vi "PH_ImageOperator.write PSDB Trace data.vi"(0 "i ref in":refnum<vi>, 5 "error in":errorcluster) -> (14 "i ref out":refnum<vi>, 15 "Trace Boolean data":T5[](array[typedef]), 16 "Trace Numeric data":T4[](array[typedef]), 17 "Trace 2D data":T3[](array[typedef]), 18 "Trace String data":T1[](array[typedef]), 19 "error out":errorcluster)   [LabVIEW 2014, in "PH_ImageOperator.lvlib"]
uses:
  PH_ImageOperator.lvlib
  PH_Basics/PH_PSDBWriter/PH_PSDBWriter.Boolean dataset.ctl
  PH_Basics/PH_PSDBWriter/PH_PSDBWriter.Numeric dataset.ctl
  PH_Basics/PH_PSDBWriter/PH_PSDBWriter.2D dataset.ctl
  CSlibraries-extern/psdb_lv/PSDB_AxisDescription.ctl
  PH_Basics/PH_PSDBWriter/PH_PSDBWriter.String dataset.ctl
  PH_Basics/PH_StatusHandler/PH_StatusHandler.Status.ctl
  CSlibraries-extern/psdb_lv/PSDB.lvlib
  PH_Basics/PH_PSDBWriter/PH_PSDBWriter.lvlib
  PH_Basics/PH_StatusHandler/PH_StatusHandler.lvlib
panel:
  in  "axis description":T2
  in  "2D data":T3
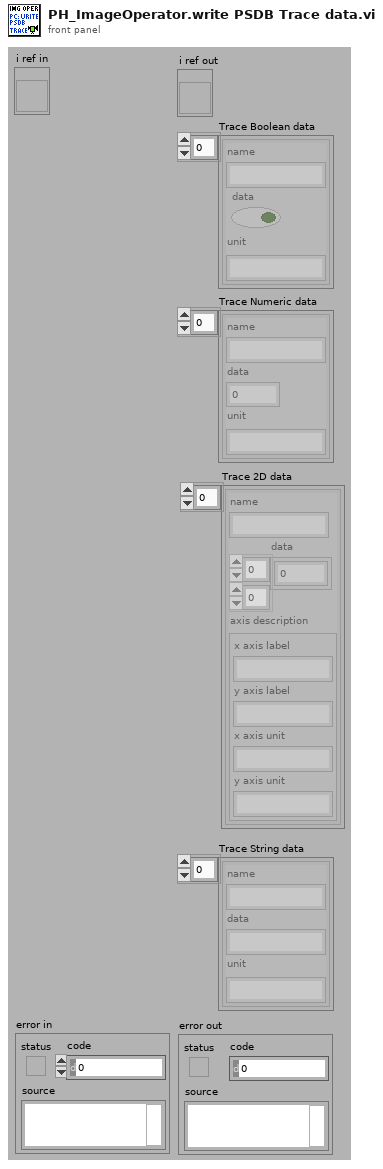
[diagram p1: front panel]
types:
  T1 = typedef "PH_PSDBWriter.lvlib/PH_PSDBWriter.String dataset.ctl" = cluster{"name":string, "data":string, "unit":string}
  T2 = typedef "PSDB.lvlib/PSDB_AxisDescription.ctl" = cluster{"x axis label":string, "y axis label":string, "x axis unit":string, "y axis unit":string}
  T3 = typedef "PH_PSDBWriter.lvlib/PH_PSDBWriter.2D dataset.ctl" = cluster{"name":string, "data":dbl[][], "axis description":T2}
  T4 = typedef "PH_PSDBWriter.lvlib/PH_PSDBWriter.Numeric dataset.ctl" = cluster{"name":string, "data":dbl, "unit":string}
  T5 = typedef "PH_PSDBWriter.lvlib/PH_PSDBWriter.Boolean dataset.ctl" = cluster{"name":string, "data":bool, "unit":string}
  T6 = typedef "PH_ImageOperator.lvlib/PH_ImageOperator.i attribute.ctl" = cluster{"GUI Refs":cluster{"Delete":refnum<vi>, "Calibration status":refnum<vi>, "BI subtracted":refnum<vi>, "calc Energy":refnum<vi>, "Energy: expected value":refnum<vi>, "Energy: Tolerance":refnum<vi>, "Energy calculated":refnum<vi>, "Energy":refnum<vi>, "calc Beam Anal":refnum<vi>, "Maj Diam 1/esquare":refnum<vi>, "Min Diam 1/esquare":refnum<vi>, "Azi Angle":refnum<vi>, "Min/Maj Diam esquare":refnum<vi>, "Beam analysed":refnum<vi>, "CoG - x":refnum<vi>, "CoG - y":refnum<vi>, "BA: Method":refnum<vi>, "BA: Steps":refnum<vi>, "BA: Factor":refnum<vi>, "calc Traces":refnum<vi>, "Traces: Fit Gauss":refnum<vi>, "Traces calculated":refnum<vi>, "Maj FWHM":refnum<vi>, "Min FWHM":refnum<vi>, "Major Trace":refnum<vi>, "Minor Trace":refnum<vi>, "Maj Fit Order":refnum<vi>, "Min Fit Order":refnum<vi>, "Position calculated":refnum<vi>, "Position":refnum<vi>, "Type":refnum<vi>, "Center":refnum<vi>, "exp - X":refnum<vi>, "exp - Y":refnum<vi>, "Tolerance":refnum<vi>, "f":refnum<vi>, "M":refnum<vi>, "D":refnum<vi>, "q":refnum<vi>, "Dummy Method":refnum<vi>, "Dummy Type":refnum<vi>, "Global On":refnum<vi>, "Traces: No offset":refnum<vi>, "Maj 99%":refnum<vi>, "Min 99%":refnum<vi>, "GUI FF Image":refnum<vi>, "calc Fill Factor":refnum<vi>, "FF calculated":refnum<vi>, "Fill Factor: Filter?":refnum<vi>, "FF: Damage Threshold":refnum<vi>, "FF: Threshold":refnum<vi>, "FF: max allow. Energy":refnum<vi>, "FF: Fillfactor":refnum<vi>, "Calibration data":refnum<vi>}, "List of GUIs":string[], "Calibration":cluster{"Status":T7, "Calibration data":T8, "Calibration Data File":path}, "Final Image":cluster{"BI Subtraction Failure":bool}, "Energy":cluster{"on":bool, "expected value [mJ]":dbl, "Tolerance [%]":dbl, "State":T7, "Energy [mJ]":dbl, "Unit":string, "calculated @":timestamp}, "Beam Analysis":cluster{"on":bool, "Data":T9, "Method":bool, "Steps":i32, "Factor":i32, "ROI":cluster{"Left":i32, "Top":i32, "Right":i32, "Bottom":i32}, "analysed @":timestamp}, "Trace Analysis":cluster{"on":bool, "Fit on":bool, "Maj FWHM":dbl, "Min FWHM":dbl, "Maj Fit Order":i32, "Min Fit Order":i32, "No Offset":bool, "Maj 99%":dbl, "Min 99%":dbl, "Traces":cluster{"XScaleName":string, "Y Scale Minimum":sgl, "Y Scale Maximum":sgl, "X Scale Minimum":sgl, "X Scale Maximum":sgl, "Traces":cluster{"Index":sgl[], "Trace":dbl[]}[]}[], "analysed @":timestamp}, "Position Analysis":cluster{"on":bool, "exp - X":i32, "exp - Y":i32, "focal length [mm]":dbl, "Magnification":dbl, "Delta":dbl, "Theta":dbl, "Tolerance":dbl, "Type":bool, "analysed @":timestamp}, "Fill Factor":cluster{"on":bool, "Filter on?":bool, "Threshold":dbl, "Damage Threshold [J/cm²]":dbl, "Fillfactor":dbl, "Max. allowed Energy [J]":dbl, "calculated @":timestamp}, "Statistician Service ID":i32, "Images":cluster{"Background":T10, "OP":T10, "GUI":T10, "BA: ROI":T10, "Trace: Turn":T10, "FF: Main":T10, "FF: Help":T10, "PSDB: BG":T10, "PSDB: OP":T10, "PSDB: FF":T10}}
  T7 = typedef "PH_StatusHandler.lvlib/PH_StatusHandler.Status.ctl" = i16
  T8 = typedef "PH_ImageCalibrator.lvlib/PH_ImageCalibrator.Calibration Data.ctl" = cluster{"Date":string, "Time":string, "Cam Settings":cluster{"Cam ID":string, "Gain":dbl, "Brightness":dbl, "Shutter":dbl, "Cam Error":bool, "Mode":i32}, "Background Image":cluster{"Image":dbl[][], "Image Error":bool}, "Linear Calibration":cluster{"Calibration Factor":dbl, "not mm or mrad":bool}, "Energy Calibration":cluster{"Calibration Factor":dbl, "no mJ":bool}}
  T9 = typedef "PH_ImageOperator.lvlib/PH_ImageOperator.Beam Analysis Data.ctl" = cluster{"CoG-x":sgl, "CoG-y":sgl, "Maj Dim":dbl, "Min Dim":dbl, "Ellipticity":dbl, "Azimuth Angle [rad]":dbl, "Azi Angle rel to Maj?":bool}
  T10 = typedef "IMAQ Image.ctl" = refnum<image>
  T11 = cluster{"XScaleName":string, "Y Scale Minimum":sgl, "Y Scale Maximum":sgl, "X Scale Minimum":sgl, "X Scale Maximum":sgl, "Traces":cluster{"Index":sgl[], "Trace":dbl[]}[]}[]
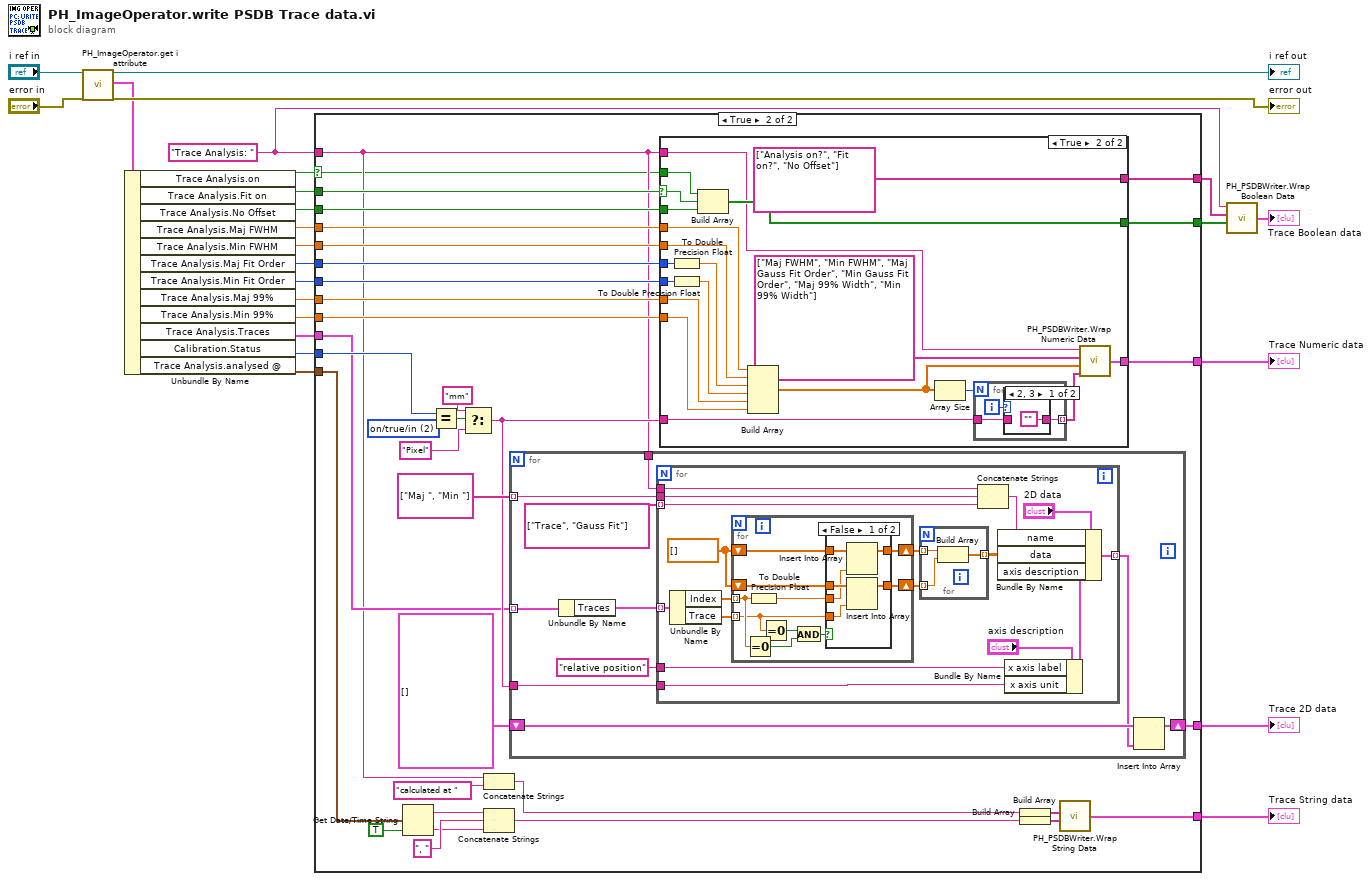
[diagram p0: block diagram]
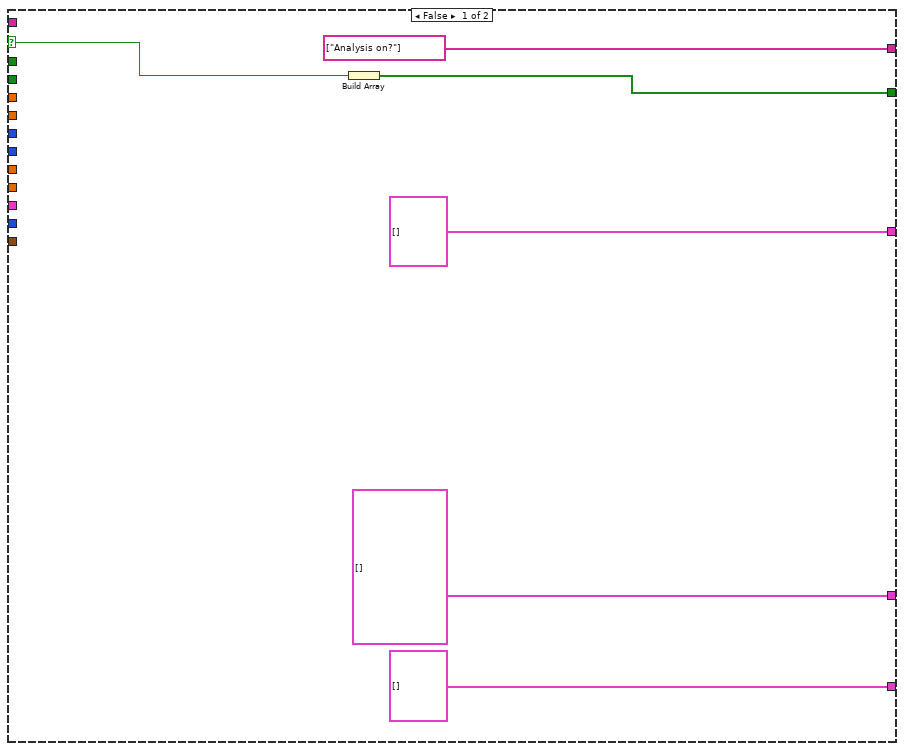
[diagram p2: hidden frame]
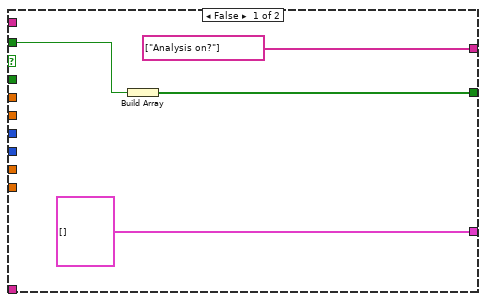
[diagram p3: hidden frame]
diagram:
  w2 = "Trace Analysis: " ("string")
  n1 = call "PH_ImageOperator.get i attribute.vi"("i ref in"="i ref in", "error in (no error)"="error in") -> ("i ref out"=→"i ref out":refnum<vi>, "i attribute"=w14:T6, "error out"=→"error out":errorcluster)  [unwired: 15 in]
  n2 = Unbundle By Name(w14) -> ("Trace Analysis.on"=w8:bool, "Trace Analysis.Fit on"=w7:bool, "Trace Analysis.No Offset"=w9:bool, "Trace Analysis.Maj FWHM"=w20:dbl, "Trace Analysis.Min FWHM"=w19:dbl, "Trace Analysis.Maj Fit Order"=w18:i32, "Trace Analysis.Min Fit Order"=w17:i32, "Trace Analysis.Maj 99%"=w16:dbl, "Trace Analysis.Min 99%"=w15:dbl, "Trace Analysis.Traces"=w12:T11, "Calibration.Status"=w13:T7, "Trace Analysis.analysed @"=w6:timestamp)
  n3 = case shown="True" w8 {
    selector: w8 -> [w26 w37]
    tunnel: w20 -> [_ w64]
    tunnel: w19 -> [_ w63]
    tunnel: w18 -> [_ w62]
    tunnel: w17 -> [_ w61]
    tunnel: w16 -> [_ w60]
    tunnel: w15 -> [_ w59]
    tunnel: w13 -> [_ w58]
    tunnel: w12 -> [_ w40]
    tunnel: [T3[] [] ("Trace 2D data") w52] -> w11
    tunnel: [T4[] [] w49] -> w10
    tunnel: w9 -> [_ w48]
    tunnel: w7 -> [_ w47]
    tunnel: w6 -> [_ w42]
    tunnel: [T1[] [] w33] -> w5
    tunnel: w2 -> [_ w39]
    tunnel: [w25 w38] -> w4
    tunnel: [string[] ["Analysis on?"] w36] -> w3
    frame False {
      n4 = Build Array(w26) -> (w25:bool[])
    }
    frame True {
      w57 = T7 2 items=["no info", "off/false/out", "on/true/in", "Failure", "Alarm", "Status 1", "Status 2", "Status 3"] ("Calibration.Status")
      n5 = Get Date/Time String(seconds (now)=w42, want seconds? (F)=TRUE) -> (date string=w45:string, time string=w43:string)  [unwired: 1 in]
      n6 = Equal?(x=w58, y=w57) -> (x = y?=w56:bool)
      n7 = Select(t="mm" ("string"), s=w56, f="Pixel" ("string")) -> (s? t:f=w50:string)
      n8 = Concatenate Strings(w39, "calculated at " ("string")) -> (w34:string)
      n9 = Concatenate Strings(w45, ", " ("string"), w43) -> (w35:string)
      n10 = for {
        tunnel: w39 -> [w103]
        tunnel: string[] ["Maj ", "Min "] -> [w102] mode=indexing
        shift-right: [w99] -> w52
        shift-left: T3[] [] ("Trace 2D data") -> [w100]
        tunnel: w50 -> [w97]
        tunnel: w40 -> [w95] mode=indexing
        n11 = Unbundle By Name(w95) -> ("Traces"=w94:cluster{"Index":sgl[], "Trace":dbl[]}[])
        n12 = for {
          tunnel: w103 -> [w120]
          tunnel: w102 -> [w119]
          tunnel: string[] ["Trace", "Gauss Fit"] -> [w118] mode=indexing
          tunnel: [w116] -> w98 mode=indexing
          tunnel: w97 -> [w112]
          tunnel: "relative position" ("x axis label") -> [w111]
          tunnel: w94 -> [w108] mode=indexing
          w107 = dbl[] []
          n13 = Unbundle By Name(w108) -> ("Index"=w109:sgl[], "Trace"=w110:dbl[])
          n14 = for {
            tunnel: w110 -> [w125] mode=indexing
            tunnel: w109 -> [w133] mode=indexing
            shift-right: [w130] -> w105
            shift-left: w107 -> [w129]
            shift-right: [w127] -> w106
            shift-left: w107 -> [w126]
            n15 = Equal To 0?(x=w133) -> (x = 0?=w131:bool)
            n16 = To Double Precision Float(number=w133) -> (double precision float=w128:dbl)
            n17 = Equal To 0?(x=w125) -> (x = 0?=w132:bool)
            n18 = And(x=w132, y=w131) -> (x .and. y?=w124:bool)
            n19 = case shown="False" w124 {
              tunnel: [w139 w140] -> w130
              tunnel: w129 -> [w138 w140]
              tunnel: w128 -> [w134 _]
              tunnel: [w137 w141] -> w127
              tunnel: w126 -> [w136 w141]
              tunnel: w125 -> [w135 _]
              frame False {
                n20 = Insert Into Array(array=w138, new element=w134) -> (w139:dbl[])  [unwired: 1 in]
                n21 = Insert Into Array(array=w136, new element=w135) -> (w137:dbl[])  [unwired: 1 in]
              }
              frame True {
              }
            }
          }
          n22 = for {
            tunnel: w106 -> [w121] mode=indexing
            tunnel: w105 -> [w122] mode=indexing
            tunnel: [w123] -> w104 mode=indexing
            n23 = Build Array(w122, w121) -> (w123:dbl[])
          }
          n24 = Concatenate Strings(w120, w119, w118) -> (w117:string)
          n25 = Bundle By Name(cluster="axis description", "x axis label"=w111, "x axis unit"=w112) -> (w113:T2)
          n26 = Bundle By Name(cluster="2D data", "name"=w117, "data"=w104, "axis description"=w113) -> (w116:T3)
        }
        n27 = Insert Into Array(array=w100, new element=w98) -> (w99:T3[])  [unwired: 1 in]
      }
      n28 = case shown="True" w47 {
        selector: w47 -> [_ w75]
        tunnel: w64 -> [_ w86]
        tunnel: w63 -> [_ w85]
        tunnel: w62 -> [_ w84]
        tunnel: w61 -> [_ w83]
        tunnel: w60 -> [_ w82]
        tunnel: w59 -> [_ w81]
        tunnel: w39 -> [_ w73]
        tunnel: w50 -> [_ w80]
        tunnel: [T4[] [] w70] -> w49
        tunnel: w48 -> [_ w79]
        tunnel: [w66 w78] -> w38
        tunnel: w37 -> [w67 w76]
        tunnel: [string[] ["Analysis on?"] string[] ["Analysis on?", "Fit on?", "No Offset"]] -> w36
        frame False {
          n29 = Build Array(w67) -> (w66:bool[])
        }
        frame True {
          n30 = To Double Precision Float(number=w84) -> (double precision float=w88:dbl)
          n31 = To Double Precision Float(number=w83) -> (double precision float=w87:dbl)
          n32 = Build Array(w76, w75, w79) -> (w78:bool[])
          n33 = Build Array(w86, w85, w88, w87, w82, w81) -> (w71:dbl[])
          n34 = Array Size(array=w71) -> (size(s)=w72:i32)
          n35 = for {
            N: w72 -> [_]
            tunnel: w80 -> [w90]
            tunnel: [w89] -> w69 mode=indexing
            i -> [w91]
            n36 = case shown="2, 3" w91 {
              tunnel: w90 -> [_ w93]
              tunnel: ["" w93] -> w89
              frame 2, 3 {
              }
              frame Default {
              }
            }
          }
          n37 = call "PH_PSDBWriter.Wrap Numeric Data.vi"("Unit Array"=w69, "Data Array"=w71, "Name Array"=string[] ["Maj FWHM", "Min FWHM", "Maj Gauss Fit Order", "Min Gauss Fit Order", "Maj 99% Width", "Min 99% Width"], "Name Prefix"=w73) -> ("PSDB Numeric Data Array"=w70:T4[])
        }
      }
      n38 = Build Array(w34) -> (w32:string[])
      n39 = Build Array(w35) -> (w31:string[])
      n40 = call "PH_PSDBWriter.Wrap String Data.vi"("Data Array"=w31, "Name Array"=w32) -> ("PSDB String Data Array"=w33:T1[])  [unwired: 2 in]
    }
  }
  "Trace Numeric data" <- w10
  "Trace 2D data" <- w11
  "Trace String data" <- w5
  n41 = call "PH_PSDBWriter.Wrap Boolean Data.vi"("Data Array"=w4, "Name Array"=w3, "Name Prefix"=w2) -> ("PSDB Boolean Data Array"=→"Trace Boolean data":T5[])  [unwired: 1 in]
